vi "Player Info.vi"(11 "Defenders in":refnum<class "Defenders.lvclass">) -> (0 "Defeat Speech":string, 1 "Victory Speech":string, 2 "Name":string, 3 "Defenders out":refnum<class "Defenders.lvclass">)   [LabVIEW 2015, in "Defenders.lvclass"]
uses:
  Defenders.lvclass
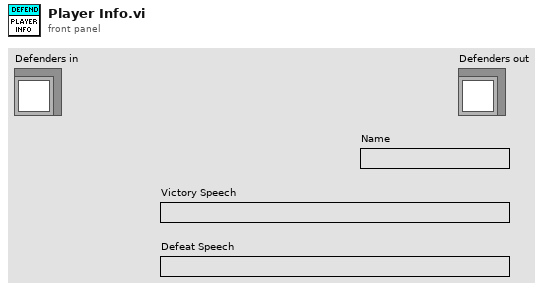
[diagram p1: front panel]
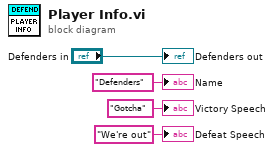
[diagram p0: block diagram]
diagram:
  "Defenders out" <- "Defenders in"
  "Name" <- "Defenders" ("Name")
  "Victory Speech" <- "Gotcha" ("Victory Speech")
  "Defeat Speech" <- "We're out" ("Defeat Speech")
